vi "Tema2.vi"() -> ()   [LabVIEW 2018]
uses:
  <vilib>/vision/NI_Vision_Development_Module.lvlib
panel:
  out "Imagine scalata":T1(plugin-control)
  out "Imagine originala":T1(plugin-control)
  in  "KxK":dbl=5.0
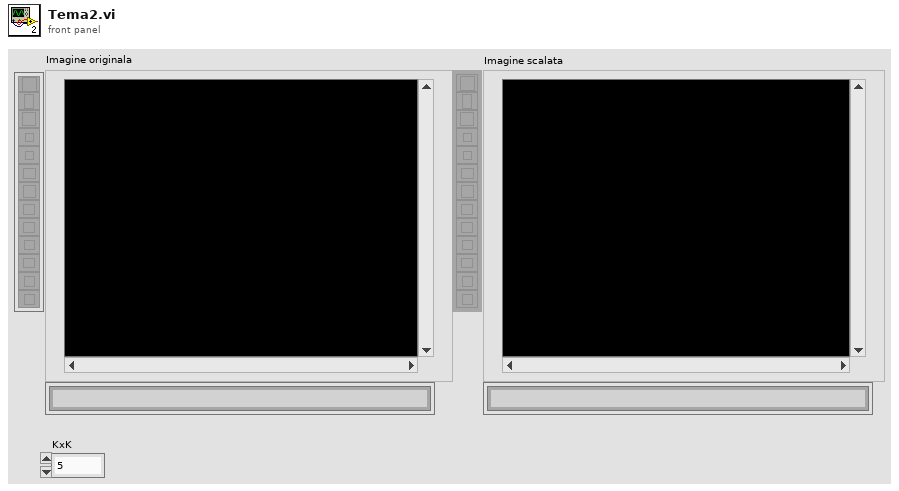
[diagram p1: front panel]
types:
  T1 = typedef "IMAQ Image.ctl" = refnum<image>
  T2 = typedef "Image Type" = u32
  T3 = cluster{"Red (or Hue) value":u8, "Green (or Sat) value":u8, "Blue (or Light or Val) value":u8}[][]
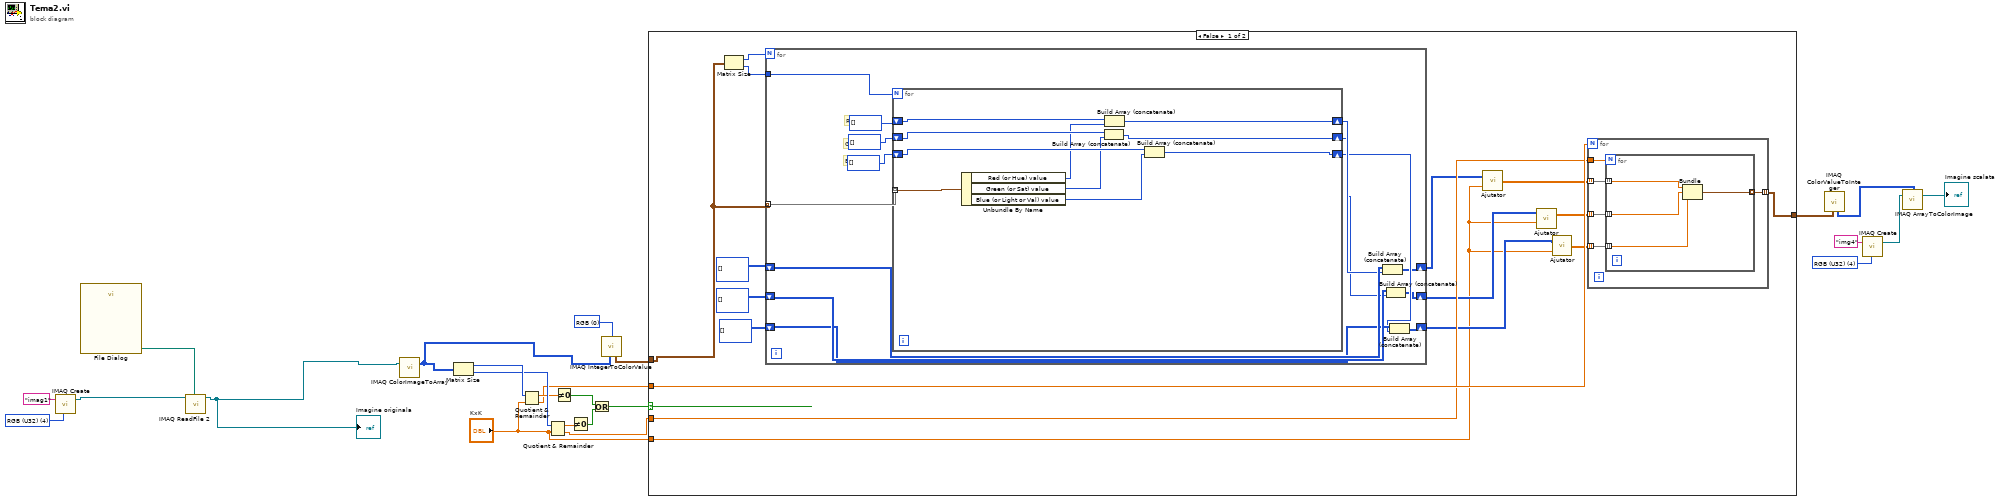
[diagram p0: block diagram]
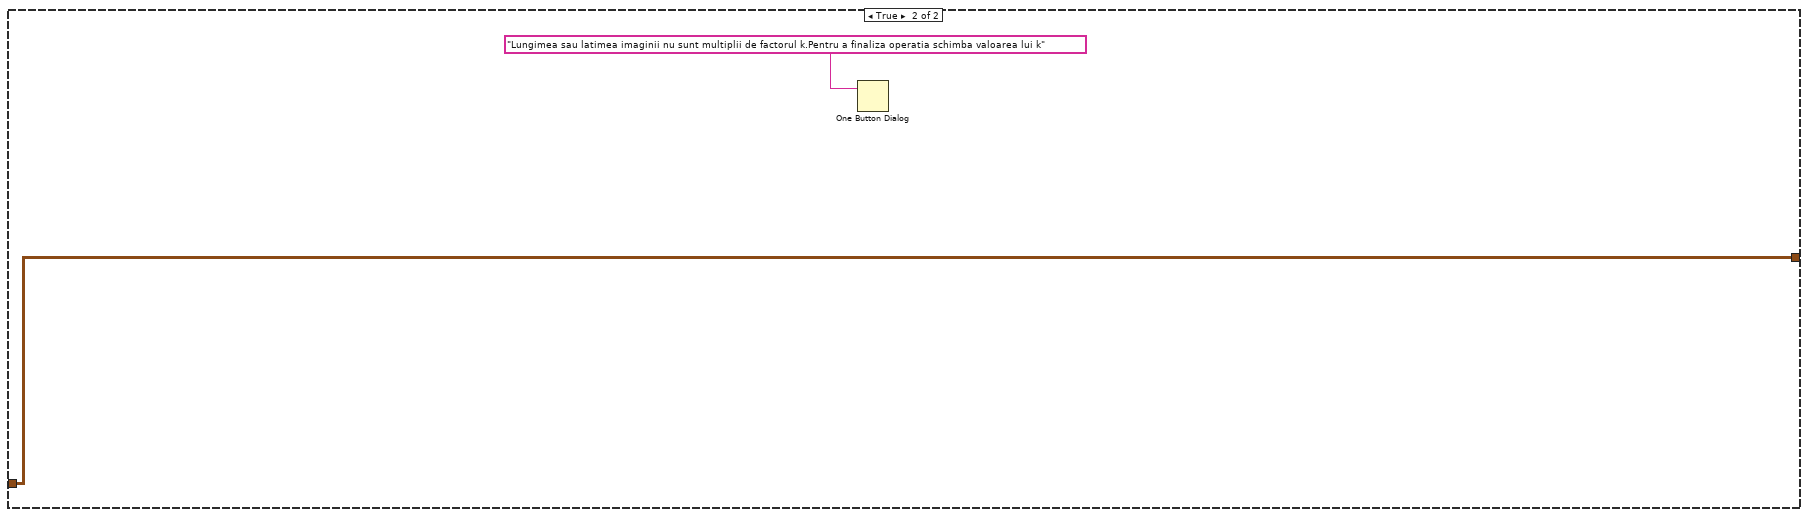
[diagram p2: hidden frame]
diagram:
  w3 = u16 0 items=["RGB", "HSL", "HSV", "HSI"] ("Color Mode")
  w9 = T2 4 items=["Grayscale (U8)", "Grayscale (I16)", "Grayscale (SGL)", "Complex (CSG)", "RGB (U32)", "HSL (U32)", "RGB (U64)", "Grayscale (U16)"] ("Image Type")
  w16 = T2 4 items=["Grayscale (U8)", "Grayscale (I16)", "Grayscale (SGL)", "Complex (CSG)", "RGB (U32)", "HSL (U32)", "RGB (U64)", "Grayscale (U16)"] ("Image Type")
  n1 = call "IMAQ Create"("Image Name"="imag1", "Image Type"=w16) -> ("New Image"=w23:T1)  [unwired: 3 in, 1 out]
  n2 = call "File Dialog"() -> ("selected path"=w22:path)  [unwired: 12 in, 3 out]
  n3 = call "IMAQ ReadFile 2"("File Path"=w22, "Image"=w23) -> ("Image Out"=w15:T1)  [unwired: 5 in, 4 out]
  "Imagine originala" <- w15
  n4 = call "IMAQ ColorImageToArray"("Image"=w15) -> ("Image Pixels (U32)"=w2:u32[][])  [unwired: 3 in, 2 out]
  n5 = Matrix Size(0:w2) -> (1:w21:i32, 2:w20:i32)
  n6 = Quotient & Remainder(x=w21, y="KxK") -> (x-y*floor(x/y)=w8:dbl, floor(x/y)=w6:dbl)
  n7 = Quotient & Remainder(x=w20, y="KxK") -> (x-y*floor(x/y)=w14:dbl, floor(x/y)=w5:dbl)
  n8 = Not Equal To 0?(x=w8) -> (x != 0?=w18:bool)
  n9 = Not Equal To 0?(x=w14) -> (x != 0?=w19:bool)
  n10 = Or(x=w18, y=w19) -> (x .or. y?=w17:bool)
  n11 = call "IMAQ IntegerToColorValue"("2D U32 array"=w2, "Color Mode"=w3) -> ("2D Color value array"=w1:T3)  [unwired: 3 in, 3 out]
  n12 = case shown="False" w17 {
    tunnel: "KxK" -> [w25 _]
    tunnel: w6 -> [w35 _]
    tunnel: w5 -> [w34 _]
    tunnel: [w33 w74] -> w4
    tunnel: w1 -> [w32 w74]
    frame False {
      n13 = Matrix Size(0:w32) -> (1:w40:i32, 2:w39:i32)
      n14 = for {
        N: w40 -> [_]
        tunnel: w32 -> [w63] mode=indexing
        tunnel: w39 -> [w62]
        shift-right: [w52] -> w30
        shift-left: i32[][] [] -> [w58]
        shift-right: [w51] -> w28
        shift-left: i32[][] [] -> [w57]
        shift-right: [w50] -> w26
        shift-left: i32[][] [] -> [w56]
        # "B"
        # "G"
        # "R"
        n15 = for {
          N: w62 -> [_]
          tunnel: w63 -> [w73] mode=indexing
          shift-right: [w66] -> w55
          shift-left: i32[] [] -> [w72]
          shift-right: [w65] -> w54
          shift-left: i32[] [] -> [w71]
          shift-right: [w64] -> w53
          shift-left: i32[] [] -> [w70]
          n16 = Unbundle By Name(w73) -> ("Red (or Hue) value"=w69:u8, "Green (or Sat) value"=w68:u8, "Blue (or Light or Val) value"=w67:u8)
          n17 = Build Array (concatenate)(w71, w68) -> (w65:i32[])
          n18 = Build Array (concatenate)(w72, w69) -> (w66:i32[])
          n19 = Build Array (concatenate)(w70, w67) -> (w64:i32[])
        }
        n20 = Build Array (concatenate)(w58, w55) -> (w52:i32[][])
        n21 = Build Array (concatenate)(w57, w54) -> (w51:i32[][])
        n22 = Build Array (concatenate)(w56, w53) -> (w50:i32[][])
      }
      n23 = call "Ajutator.vi"("kxk"=w25, "Input"=w30) -> ("Output"=w31:dbl[][])
      n24 = call "Ajutator.vi"("kxk"=w25, "Input"=w28) -> ("Output"=w29:dbl[][])
      n25 = call "Ajutator.vi"("kxk"=w25, "Input"=w26) -> ("Output"=w27:dbl[][])
      n26 = for {
        N: w35 -> [_]
        tunnel: w31 -> [w45] mode=indexing
        tunnel: w29 -> [w44] mode=indexing
        tunnel: w27 -> [w43] mode=indexing
        tunnel: [w42] -> w33 mode=indexing
        tunnel: w34 -> [w41]
        n27 = for {
          N: w41 -> [_]
          tunnel: w45 -> [w49] mode=indexing
          tunnel: w44 -> [w48] mode=indexing
          tunnel: w43 -> [w47] mode=indexing
          tunnel: [w46] -> w42 mode=indexing
          n28 = Bundle(w49, w48, w47) -> (w46:cluster{dbl, dbl, dbl})  [unwired: 1 in]
        }
      }
    }
    frame True {
      n29 = One Button Dialog(message="Lungimea sau latimea imaginii nu sunt multiplii de factorul k.Pentru a finaliza operatia schimba valoarea lui k") -> ()  [unwired: 1 in, 1 out]
    }
  }
  n30 = call "IMAQ ColorValueToInteger"("2D Color value array"=w4) -> ("2D U32 array"=w13:u32[][])  [unwired: 4 in, 3 out]
  n31 = call "IMAQ Create"("Image Name"="img4", "Image Type"=w9) -> ("New Image"=w11:T1)  [unwired: 3 in, 1 out]
  n32 = call "IMAQ ArrayToColorImage"("Image Pixels (U32)"=w13, "Image"=w11) -> ("Image Out"=→"Imagine scalata":T1)  [unwired: 3 in, 1 out]
